vi "Emisor Fortu.vi"() -> ()   [LabVIEW 2020]
uses:
  <vilib>/Instr/_visa.llb/VISA Configure Serial Port (Instr).vi
panel:
  in  "stop":bool
  out "String":string
  out "LUZ":bool
  in  "VISA resource name":refnum<visa-resource-name>
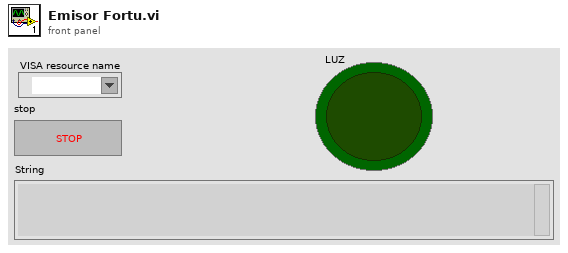
[diagram p1: front panel]
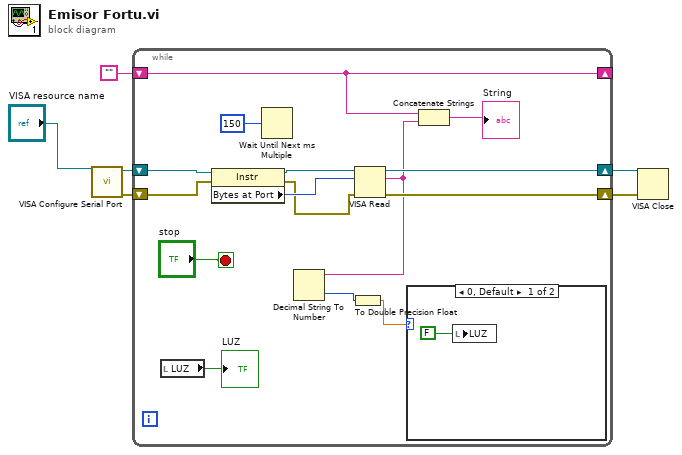
[diagram p0: block diagram]
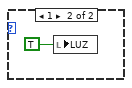
[diagram p2: hidden frame]
diagram:
  n1 = call-poly "VISA Configure Serial Port"("VISA resource name"="VISA resource name") -> ("VISA resource name out"=w6:refnum<visa-resource-name>, "error out"=w5:errorcluster)  [unwired: 13 in]
  n2 = while {
    shift-right: [w18] -> w4
    shift-left: w6 -> [w21]
    shift-right: [w17] -> w3
    shift-left: w5 -> [w20]
    shift-right: [w15] -> _
    shift-left: "" -> [w15]
    stop <- "stop" stop-if-true
    n3 = local read "LUZ"() -> (→"LUZ":bool)
    n4 = property class="Instr"(reference=w21, error in=w20) -> (reference out=w13:refnum<visa-resource-name>, error out=w12:errorcluster, "Bytes at Port"=w19:u32)
    n5 = Wait Until Next ms Multiple(millisecond multiple=u32 150 ("milliseconds to wait")) -> ()  [unwired: 1 out]
    n6 = VISA Read(VISA resource name=w13, byte count=w19, error in (no error)=w12) -> (VISA resource name out=w18:refnum<visa-resource-name>, read buffer=w11:string, error out=w17:errorcluster)  [unwired: 1 out]
    n7 = Decimal String To Number(string=w11) -> (number=w10:i32)  [unwired: 2 in, 1 out]
    n8 = To Double Precision Float(number=w10) -> (double precision float=w8:dbl)
    n9 = case shown="0, Default" w8 {
      frame 0, Default {
        n10 = local write "LUZ"(FALSE) -> ()
      }
      frame 1 {
        n11 = local write "LUZ"(TRUE) -> ()
      }
    }
    n12 = Concatenate Strings(w15, w11) -> (→"String":string)
  }
  n13 = VISA Close(VISA resource name=w4, error in (no error)=w3) -> ()  [unwired: 1 out]
